vi "Save Config.vi"(8 "error in (no error)":errorcluster, 10 "FileName":string="SerialConfig.xml", 11 "Serial Config":T1={"串口选择"="", "通讯速率"=9600, "超时时间"=10000, "数据位长"=8, "奇偶校验"=enum."None", "停止位长"=10, "握手控制"=0, "字符结束"=TRUE, "结束字符"=10} {"结束字符" format="%.0x"; "握手控制" items=["None", "XON/XOFF", "RTS/CTS", "XON/XOFF & RTS/CTS", "DTR/DSR", "XON/XOFF & DTR/DSR"]; "停止位长" items=["1.0"=10, "1.5"=15, "2.0"=20]; "数据位长" min=5 max=8 step=1}) -> (0 "error out":errorcluster)   [LabVIEW 2010, in "CenterOne.lvlib"]
doc: "Use this template to build a VI to use as a subVI."
uses:
  CenterOne.lvlib
  Serial Config.ctl
  <vilib>/Utility/xml.llb/Write to XML File(string).vi
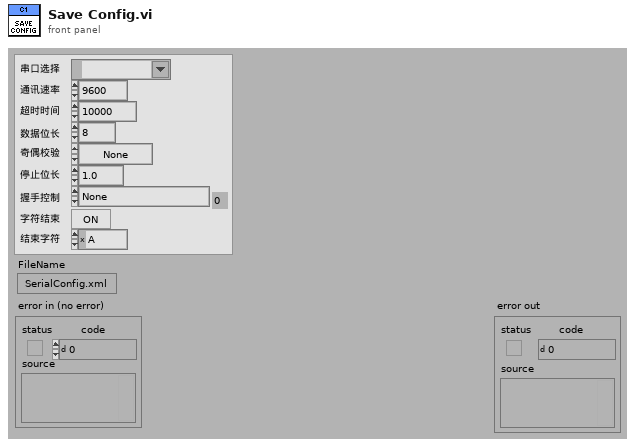
[diagram p1: front panel]
types:
  T1 = typedef "CenterOne.lvlib/Serial Config.ctl" = cluster{"串口选择":refnum<visa-resource-name>, "通讯速率":u32, "超时时间":u32, "数据位长":u16, "奇偶校验":enum16{"None", "Odd", "Even", "Mark", "Space"}, "停止位长":u16, "握手控制":u16, "字符结束":bool, "结束字符":u8}
  T2 = enum32{"invalid app kind", "Development System", "Run Time System", "Student Edition", "Embedded LabVIEW", "Evaluation", "Custom"}
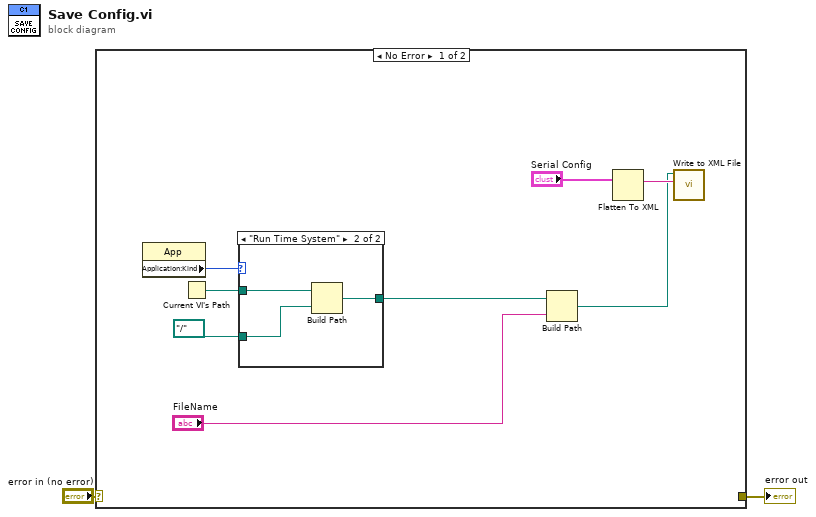
[diagram p0: block diagram]
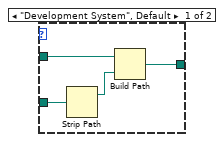
[diagram p2: hidden frame]
diagram:
  n1 = case shown="No Error" "error in (no error)" {
    selector: "error in (no error)" -> [_ w18]
    tunnel: [_ w18] -> w1
    frame No Error {
      n2 = property class="App"() -> ("Application:Kind"=w3:T2)  [unwired: 2 in, 2 out]
      n3 = Current VI's Path() -> (path=w9:path)
      n4 = case shown="\"Run Time System\"" w3 {
        tunnel: [w14 w15] -> w7
        tunnel: w9 -> [w13 w17]
        tunnel: path "../.." ("relative path (.)") -> [w12 w16]
        frame "Development System", Default {
          n5 = Strip Path(path=w12) -> (stripped path=w11:path)  [unwired: 1 out]
          n6 = Build Path(base path=w13, name or relative path=w11) -> (appended path=w14:path)
        }
        frame "Run Time System" {
          n7 = Build Path(base path=w17, name or relative path=w16) -> (appended path=w15:path)
        }
      }
      n8 = Build Path(base path=w7, name or relative path="FileName") -> (appended path=w5:path)
      n9 = Flatten To XML(anything="Serial Config") -> (xml string=w10:string)
      n10 = call-poly <vilib>:"Write to XML File.vi"("XML Input"=w10, "XML File Path"=w5) -> ()  [unwired: 7 in, 3 out]
    }
    frame Error {
    }
  }
  "error out" <- w1
